vi "TC State Machine State Transition Trace.vi"(4 "error in (no error)":errorcluster, 6 "Launch Order":i32, 7 "Next State":T1) -> (0 "error out":errorcluster)   [LabVIEW 2020, in "Startup Processes.lvlib"]
uses:
  Startup Processes.lvlib
  _typedefs/States.ctl
  toolbox/Debugging/Debugging.lvlib
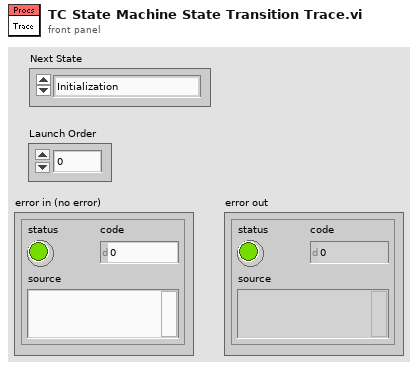
[diagram p1: front panel]
types:
  T1 = typedef "Startup Processes.lvlib/States.ctl" = enum16{"Initialization", "Read Input", "Test Fan Limits", "Set Fan", "Test Cooler Limits", "Set Cooler", "Acquisition TO Wait", "Error", "Deinitialize"}
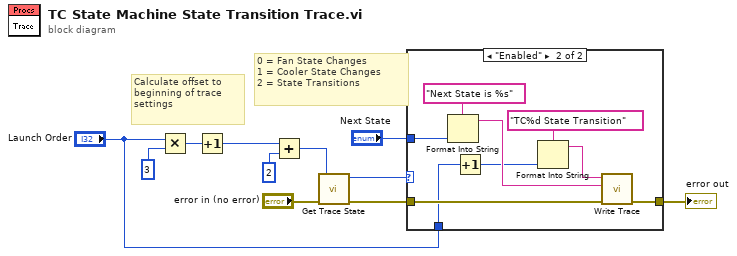
[diagram p0: block diagram]
diagram:
  # "0 = Fan State Changes\n1 = Cooler State Changes\n2 = State Transitions"
  # "Calculate offset to beginning of trace settings"
  n1 = Multiply(x="Launch Order", y=3) -> (x*y=w10:i32)
  n2 = Increment(x=w10) -> (x+1=w9:i32)
  n3 = Add(x=w9, y=2) -> (x+y=w4:i32)
  n4 = call "Get Trace State.vi"("Error In"="error in (no error)", "Trace Point Index"=w4) -> ("Error Out"=w7:errorcluster, "Trace Point State"=w6:enum16{"Disabled", "Enabled"})  [unwired: 4 in]
  n5 = case shown="\"Enabled\"" w6 {
    tunnel: w7 -> [w12 w21]
    tunnel: [w12 w20] -> w5
    tunnel: "Next State" -> [_ w19]
    tunnel: "Launch Order" -> [_ w14]
    frame "Disabled" {
    }
    frame "Enabled" {
      n6 = Format Into String(format string="Next State is %s", w19) -> (resulting string=w18:string)  [unwired: 2 in, 1 out]
      n7 = Increment(x=w14) -> (x+1=w13:i32)
      n8 = Format Into String(format string="TC%d State Transition" ("Trace Point Name"), w13) -> (resulting string=w16:string)  [unwired: 2 in, 1 out]
      n9 = call "Write Trace.vi"("Error In"=w21, "Trace Data"=w18, "Trace Point Name"=w16) -> ("Error Out"=w20:errorcluster)  [unwired: 4 in]
    }
  }
  "error out" <- w5
